vi "Parse elements.vi"(0 "Is array?":bool, 1 "Non indexed arrays?":bool, 3 "Required object":string, 5 "Single path element":string, 7 "Complete Array?":bool, 9 "JSON Path":string, 11 "error in (no error)":errorcluster, 12 "Variant":variant, 13 "Array contained cluster?":bool) -> (6 "VArray":variant, 15 "error out":errorcluster)   [LabVIEW 2015]
uses:
  <vilib>/Utility/Data Type/Type Definitions/Data Type.ctl
  <vilib>/Utility/Data Type/NI_Data Type.lvlib
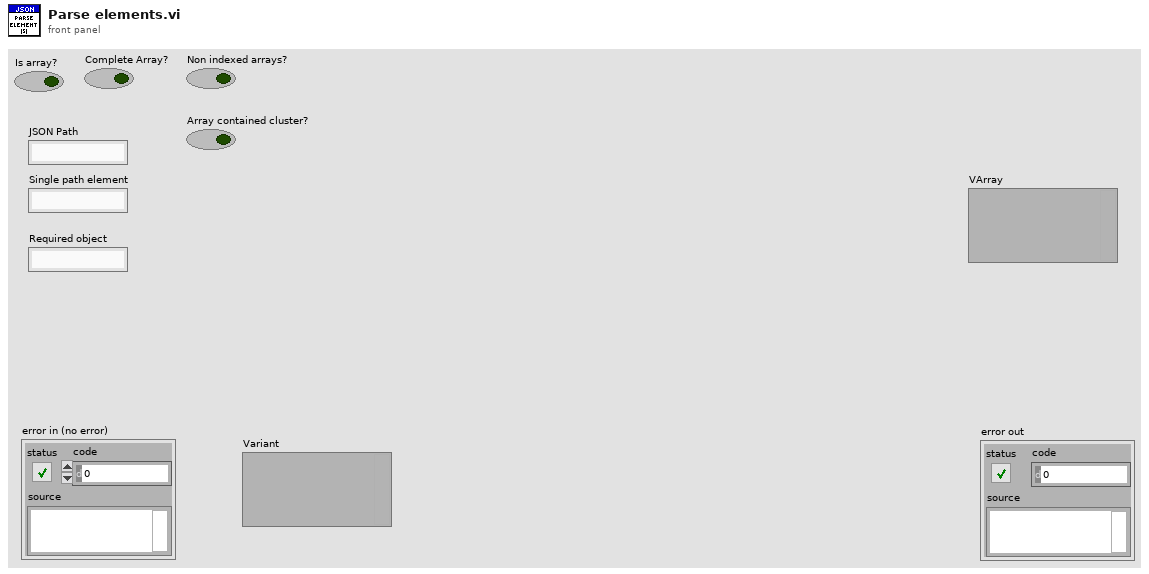
[diagram p1: front panel]
types:
  T1 = typedef "NI_Data Type.lvlib/Data Type.ctl" = enum8{"Invalid Type", "Void", "I8", "I16", "I32", "I64", "U8", "U16", "U32", "U64", "Single Float", "Double Float", "Extended Float", "Single Complex", "Double Complex", "Extended Complex", "Enum U8", "Enum U16", "Enum U32", "Enum U64", "Single Float With Unit", "Double Float With Unit", "Extended Float With Unit", "Single Complex with Unit", "Double Complex with Unit", "Extended Complex with Unit", "Boolean", "String", "Path", "Picture", "Tag", "Array", "Cluster", "Variant", "LV Variant", "Waveform", "Timestamp", "Digital Waveform", "Digital Data", "ExpressData", "Refnum", "External Data", "VI", "Poly VI", "LabVIEW Class Instance", "Fixed Point"}
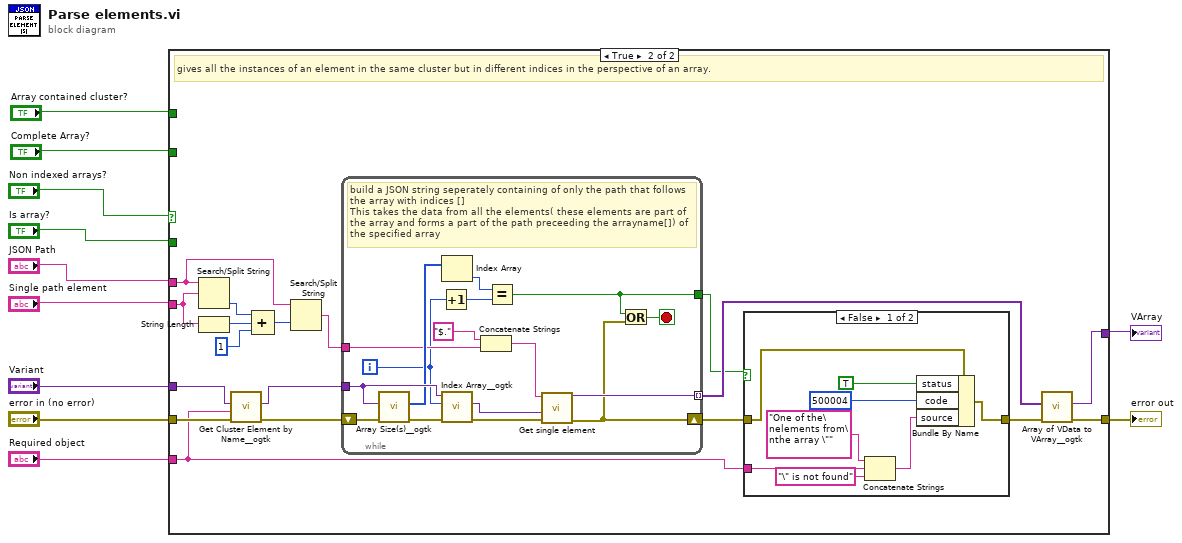
[diagram p0: block diagram]
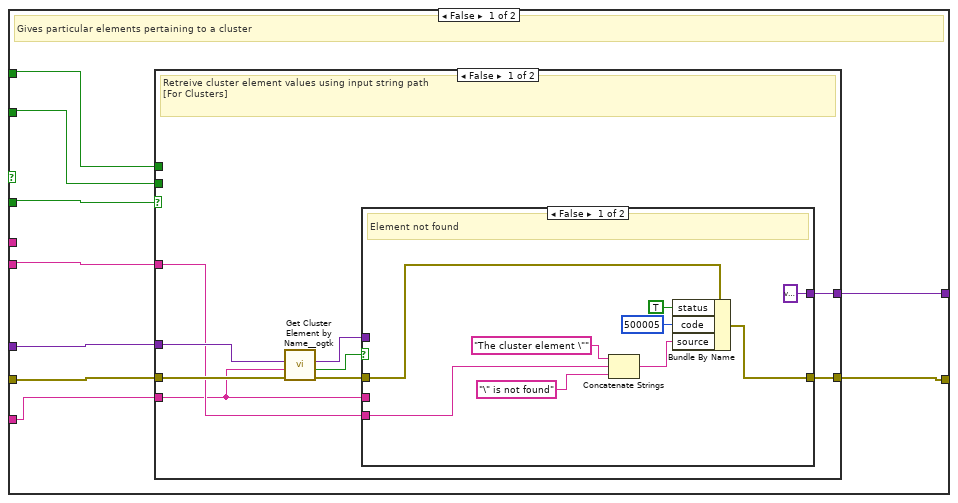
[diagram p2: hidden frame]
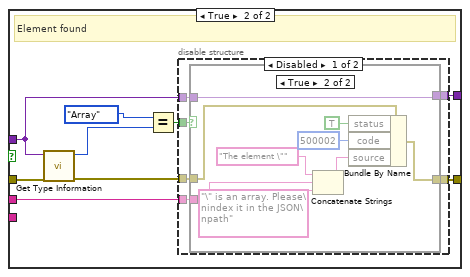
[diagram p3: hidden frame]
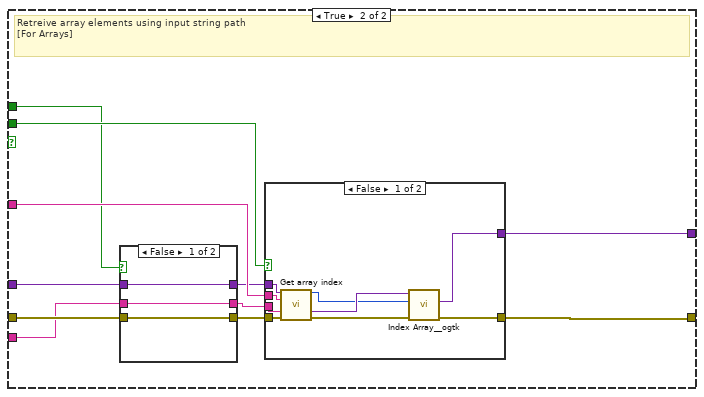
[diagram p6: hidden frame]
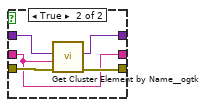
[diagram p7: hidden frame]
diagram:
  n1 = case shown="True" "Non indexed arrays?" {
    tunnel: [w20 w113] -> w8
    tunnel: "error in (no error)" -> [w19 w108]
    tunnel: [w18 w112] -> w4
    tunnel: "Required object" -> [w17 w104]
    tunnel: "Single path element" -> [w16 w101]
    tunnel: "Is array?" -> [w15 _]
    tunnel: "Variant" -> [w14 w106]
    tunnel: "JSON Path" -> [_ w99]
    tunnel: "Complete Array?" -> [w13 _]
    tunnel: "Array contained cluster?" -> [w12 _]
    frame False {
      # "Gives particular elements pertaining to a cluster"
      n2 = case shown="False" w15 {
        tunnel: w14 -> [w29 w73]
        tunnel: [w24 w75] -> w20
        tunnel: w16 -> [w22 w77]
        tunnel: w19 -> [w28 w72]
        tunnel: [w26 w76] -> w18
        tunnel: w17 -> [w21 w70]
        tunnel: w13 -> [_ w74]
        tunnel: w12 -> [_ w67]
        frame False {
          # "Retreive cluster element values using input string path\n[For Clusters]"
          n3 = call <userlib>:"Get Cluster Element by Name__ogtk.vi"("error in (no error)"=w28, "Element Name"=w21, "Cluster"=w29) -> ("error out"=w27:errorcluster, "found?"=w23:bool, "VElement"=w25:variant)  [unwired: 6 in]
          n4 = case shown="False" w23 {
            tunnel: w27 -> [w38 w47]
            tunnel: w21 -> [_ w44]
            tunnel: [w31 w41] -> w26
            tunnel: w25 -> [_ w40]
            tunnel: [variant ("VElement") w39] -> w24
            tunnel: w22 -> [w34 _]
            frame False {
              # "Element not found"
              n5 = Concatenate Strings("The cluster element \"" ("source"), w34, "\" is not found" ("string")) -> (w32:string)
              n6 = Bundle By Name(cluster=w38, "status"=TRUE, "code"=500005, "source"=w32) -> (w31:errorcluster)
            }
            frame True {
              # "Element found"
              n7 = call <vilib>:"Get Type Information.vi"("error in (no error)"=w47, "Variant"=w40) -> ("error out"=w42:errorcluster, "Type"=w46:T1)  [unwired: 5 in, 3 out]
              n8 = Equal?(x=Data_Type."Array", y=w46) -> (x = y?=w43:bool)
              n9 = disable-structure shown="Disabled" {
                disable-tunnel: w44 -> [w53 _]
                disable-tunnel: w43 -> [w52 _]
                disable-tunnel: w42 -> [w51 w65]
                disable-tunnel: [w50 w65] -> w41
                disable-tunnel: w40 -> [w49 w66]
                disable-tunnel: [w48 w66] -> w39
                frame Disabled {
                  n10 = case shown="True" w52 {
                    tunnel: w53 -> [_ w60]
                    tunnel: w51 -> [w55 w64]
                    tunnel: [w55 w57] -> w50
                    tunnel: w49 -> [w54 w56]
                    tunnel: [w54 w56] -> w48
                    frame False {
                    }
                    frame True {
                      n11 = Concatenate Strings("The element \"" ("source"), w60, "\" is an array. Please\nindex it in the JSON\npath" ("string")) -> (w58:string)
                      n12 = Bundle By Name(cluster=w64, "status"=TRUE, "code"=500002, "source"=w58) -> (w57:errorcluster)
                    }
                  }
                }
                frame Enabled {
                }
              }
            }
          }
        }
        frame True {
          # "Retreive array elements using input string path\n[For Arrays]"
          n13 = case shown="False" w67 {
            tunnel: w73 -> [w78 w85]
            tunnel: w72 -> [w80 w84]
            tunnel: [w80 w83] -> w71
            tunnel: w70 -> [w79 w81]
            tunnel: [w79 w81] -> w69
            tunnel: [w78 w82] -> w68
            frame False {
            }
            frame True {
              n14 = call <userlib>:"Get Cluster Element by Name__ogtk.vi"("error in (no error)"=w84, "Element Name"=w81, "Cluster"=w85) -> ("error out"=w83:errorcluster, "VElement"=w82:variant)  [unwired: 6 in, 1 out]
            }
          }
          n15 = case shown="False" w74 {
            tunnel: w71 -> [w93 w95]
            tunnel: w68 -> [w92 w96]
            tunnel: w77 -> [w91 _]
            tunnel: [w90 w95] -> w76
            tunnel: [w89 w96] -> w75
            tunnel: w69 -> [w86 _]
            frame False {
              n16 = call "Get array index.vi"("Variant in"=w92, "brackettedElements"=w91, "requriedObject"=w86, "error in (no error)"=w93) -> ("indexOut"=w87:i32, "VArray"=w94:variant, "error out"=w88:errorcluster)  [unwired: 5 in, 4 out]
              n17 = call <userlib>:"Index Array__ogtk.vi"("error in (no error)"=w88, "Index (1D)"=w87, "MultiD Array"=w94) -> ("error out"=w90:errorcluster, "Array Element"=w89:variant)  [unwired: 7 in]
            }
            frame True {
            }
          }
        }
      }
    }
    frame True {
      # "gives all the instances of an element in the same cluster but in different indices in the perspective of an array."
      n18 = Search/Split String(string=w99, search string/char (-)=w101) -> (offset of match=w103:i32)  [unwired: 1 in, 2 out]
      n19 = String Length(string=w101) -> (length=w102:i32)
      n20 = call <userlib>:"Get Cluster Element by Name__ogtk.vi"("error in (no error)"=w108, "Element Name"=w104, "Cluster"=w106) -> ("error out"=w107:errorcluster, "VElement"=w105:variant)  [unwired: 6 in, 1 out]
      n21 = Compound Arithmetic op=ADD(w103, w102, 1 ("value")) -> (w98:i32)
      n22 = Search/Split String(string=w99, offset (0)=w98) -> (match + rest of string=w97:string)  [unwired: 1 in, 2 out]
      n23 = while {
        tunnel: w105 -> [w139]
        tunnel: w97 -> [w135]
        tunnel: [w129] -> w114 mode=indexing
        tunnel: [w127] -> w109
        shift-right: [w128] -> w110
        shift-left: w107 -> [w132]
        i -> [w134]
        stop <- w126 stop-if-true
        # "build a JSON string seperately containing of only the path that follows the array with indices []\nThis takes the data from all the elements( these elements are part of the array and forms a part of the path preceeding the arrayname[]) of the specified array"
        n24 = call <userlib>:"Array Size(s)__ogtk.vi"("error in (no error)"=w132, "Array"=w139) -> ("error out"=w131:errorcluster, "Size(s)"=w138:u32[])  [unwired: 7 in, 1 out]
        n25 = Increment(x=w134) -> (x+1=w133:i32)
        n26 = Index Array(array=w138) -> (element=w137:u32)  [unwired: 1 in]
        n27 = call <userlib>:"Index Array__ogtk.vi"("error in (no error)"=w131, "Index (1D)"=w134, "MultiD Array"=w139) -> ("error out"=w124:errorcluster, "Array Element"=w125:variant)  [unwired: 7 in]
        n28 = Concatenate Strings("$." ("string"), w135) -> (w130:string)
        n29 = Equal?(x=w137, y=w133) -> (x = y?=w127:bool)
        n30 = call "Get single element.vi"("error in (no error)"=w124, "Variant in"=w125, "String"=w130) -> ("error out"=w128:errorcluster, "Variant out"=w129:variant)  [unwired: 7 in]
        n31 = Or(x=w127, y=w128) -> (x .or. y?=w126:bool)
      }
      n32 = case shown="False" w109 {
        tunnel: [w116 w123] -> w111
        tunnel: w110 -> [w122 w123]
        tunnel: w104 -> [w118 _]
        frame False {
          n33 = Concatenate Strings("One of the\nelements from\nthe array \"" ("source"), w118, "\" is not found" ("string")) -> (w115:string)
          n34 = Bundle By Name(cluster=w122, "status"=TRUE, "code"=500004, "source"=w115) -> (w116:errorcluster)
        }
        frame True {
        }
      }
      n35 = call <userlib>:"Array of VData to VArray__ogtk.vi"("error in (no error)"=w111, "1D Array of VData"=w114) -> ("error out"=w112:errorcluster, "VArray"=w113:variant)  [unwired: 8 in]
    }
  }
  "VArray" <- w8
  "error out" <- w4
